vi "POST data sender.vi"() -> ()   [LabVIEW 2016]
uses:
  <vilib>/httpClient/POSTBuffer.vi
  <vilib>/httpClient/LabVIEWHTTPClient.lvlib
panel:
  in  "buffer":string="Addr=00AA11BBCCDE&Temp=23.7&Hum=65.5"
  out "body":string
  out "headers":string
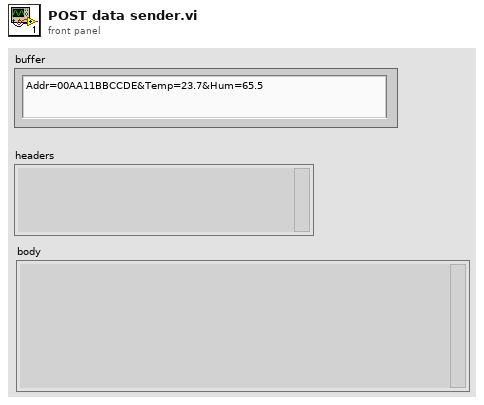
[diagram p1: front panel]
types:
  T1 = typedef "LabVIEWHTTPClient.lvlib/ClientHandle.ctl" = refnum<k1>
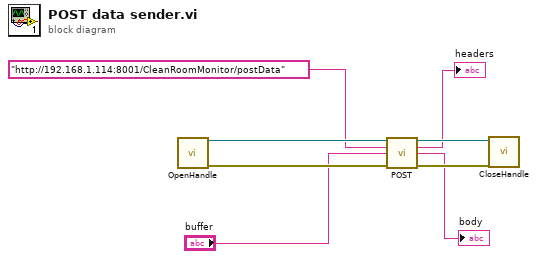
[diagram p0: block diagram]
diagram:
  n1 = call <vilib>:"OpenHandle.vi"() -> ("client handle out"=w8:T1, "error out"=w5:errorcluster)  [unwired: 14 in]
  n2 = call-poly <vilib>:"POST.vi"("client handle"=w8, "url"="http://192.168.1.114:8001/CleanRoomMonitor/postData", "buffer"="buffer", "error in (no error)"=w5) -> ("client handle out"=w7:T1, "headers"=→"headers":string, "body"=→"body":string, "error out"=w6:errorcluster)  [unwired: 8 in]
  n3 = call <vilib>:"CloseHandle.vi"("client handle"=w7, "error in (no error)"=w6) -> ()  [unwired: 13 in, 1 out]
